vi "Scanner_Ansteuerung_X-Steps.vi"(8 "X-Min / [V]":dbl, 9 "X-Max / [V]":dbl, 11 "X-Pixels":u32) -> (0 "X-Array out":dbl[](array[numeric]))   [LabVIEW 2009]
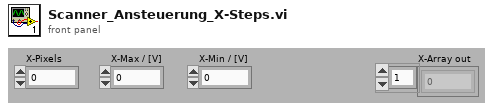
[diagram p1: front panel]
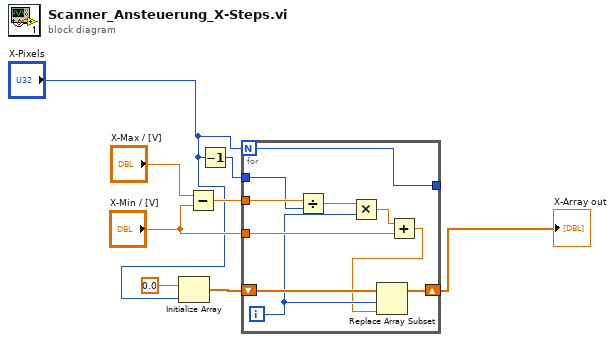
[diagram p0: block diagram]
diagram:
  n1 = Initialize Array(0.0 ("element"), "X-Pixels") -> (w4:dbl[])
  n2 = Subtract(x="X-Max / [V]", y="X-Min / [V]") -> (x-y=w7:dbl)
  n3 = Decrement(x="X-Pixels") -> (x-1=w2:u32)
  n4 = for {
    N: "X-Pixels" -> [w15]
    tunnel: w7 -> [w18]
    tunnel: "X-Min / [V]" -> [w14]
    tunnel: [w15] -> _
    tunnel: w2 -> [w13]
    shift-right: [w9] -> w3
    shift-left: w4 -> [w12]
    i -> [w11]
    n5 = Divide(x=w18, y=w13) -> (x/y=w17:dbl)
    n6 = Multiply(x=w17, y=w11) -> (x*y=w16:dbl)
    n7 = Add(x=w16, y=w14) -> (x+y=w10:dbl)
    n8 = Replace Array Subset(array=w12, new element=w10, index=w11) -> (w9:dbl[])
  }
  "X-Array out" <- w3
